vi "LinkNodes.vi"(0 "Parent in":refnum<data-value>, 5 "Child in":refnum<data-value>, 7 "ParentLinkInfo":T1, 9 "ChildLinkInfo":T1, 11 "error in (no error)":errorcluster) -> (4 "Parent out":refnum<data-value>, 6 "Child out":refnum<data-value>, 15 "error out":errorcluster)   [LabVIEW 2014, in "MultiTree.lvlib" / "MultiTree.lvclass"]
uses:
  <userlib>/AdvancedDataStructures/ClassBased/MultiTree/MultiTree.lvclass
  <userlib>/AdvancedDataStructures/ClassBased/MultiTreeNode/MultiTreeNode.lvclass
  <userlib>/AdvancedDataStructures/ClassBased/MultiTree/LinkInfo.ctl
  <userlib>/AdvancedDataStructures/ClassBased/MultiTreeNode/MultiTreeNode.lvclass/MultiTreeNode.ctl
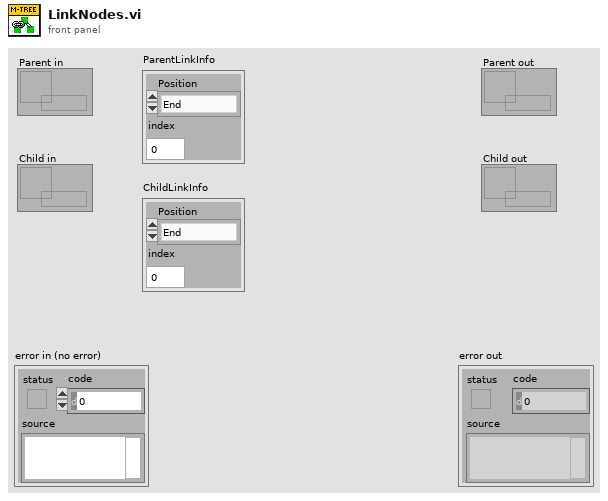
[diagram p1: front panel]
types:
  T1 = typedef "MultiTree.lvlib/MultiTree.lvclass/LinkInfo.ctl" = cluster{"Position":enum16{"End", "Front", "Index"}, "index":i32}
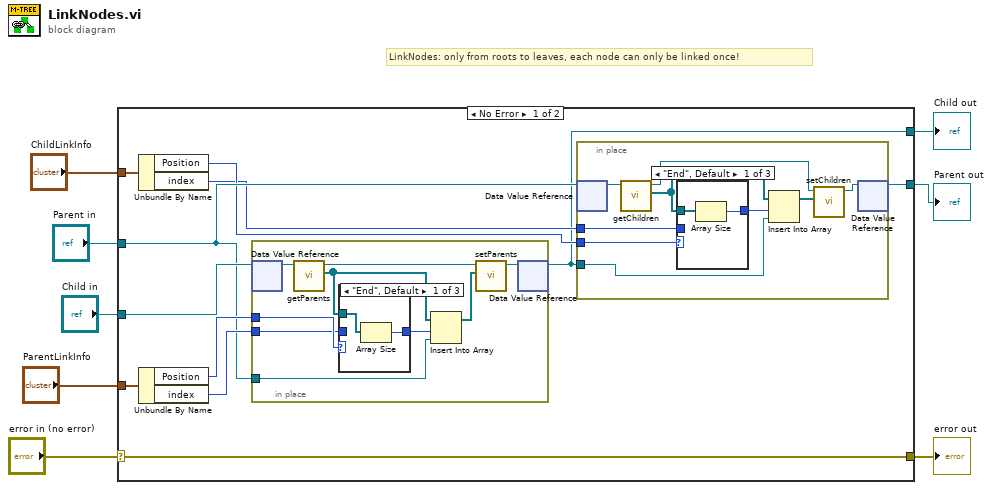
[diagram p0: block diagram]
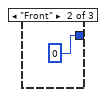
[diagram p2: hidden frame]
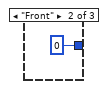
[diagram p4: hidden frame]
diagram:
  # "LinkNodes: only from roots to leaves, each node can only be linked once!"
  n1 = case shown="No Error" "error in (no error)" {
    selector: "error in (no error)" -> [w19 w48]
    tunnel: [w19 w48] -> w7
    tunnel: "Child in" -> [w15 w46]
    tunnel: [w10 w47] -> w4
    tunnel: "Parent in" -> [w13 w47]
    tunnel: [w9 w46] -> w3
    tunnel: "ParentLinkInfo" -> [w18 _]
    tunnel: "ChildLinkInfo" -> [w17 _]
    frame No Error {
      n2 = Unbundle By Name(w17) -> ("Position"=w12:enum16{"End", "Front", "Index"}, "index"=w11:i32)
      n3 = Unbundle By Name(w18) -> ("Position"=w16:enum16{"End", "Front", "Index"}, "index"=w14:i32)
      n4 = in-place {
        in-place-border: w16 -> [w41]
        in-place-border: w14 -> [w36]
        in-place-border: w13 -> [w33]
        n5 = in-place-dvr #1(w15) -> (w40:refnum<class "MultiTreeNode.lvclass">)  [unwired: 1 out]
        n6 = call <userlib>:"getParents.vi"("MultiTreeNode in"=w40) -> ("Parents"=w35:refnum<data-value>[], "MultiTreeNode out"=w39:refnum<class "MultiTreeNode.lvclass">)  [unwired: 8 in, 1 out]
        n7 = case shown="\"End\", Default" w41 {
          tunnel: [w42 0 w45] -> w34
          tunnel: w36 -> [_ _ w45]
          tunnel: w35 -> [w43 _ _]
          frame "End", Default {
            n8 = Array Size(array=w43) -> (size(s)=w42:i32)
          }
          frame "Front" {
          }
          frame "Index" {
          }
        }
        n9 = Insert Into Array(array=w35, index=w34, new element=w33) -> (w37:refnum<data-value>[])
        n10 = call <userlib>:"setParents.vi"("Parents"=w37, "MultiTreeNode in"=w39) -> ("MultiTreeNode out"=w38:refnum<class "MultiTreeNode.lvclass">)  [unwired: 8 in, 1 out]
        n11 = in-place-dvr #1(w38) -> (w9:refnum<data-value>)  [unwired: 1 out]
      }
      n12 = in-place {
        in-place-border: w12 -> [w28]
        in-place-border: w11 -> [w23]
        in-place-border: w9 -> [w20]
        n13 = in-place-dvr #2(w13) -> (w27:refnum<class "MultiTreeNode.lvclass">)  [unwired: 1 out]
        n14 = call <userlib>:"getChildren.vi"("MultiTreeNode in"=w27) -> ("Children"=w22:refnum<data-value>[], "MultiTreeNode out"=w26:refnum<class "MultiTreeNode.lvclass">)  [unwired: 8 in, 1 out]
        n15 = case shown="\"End\", Default" w28 {
          tunnel: [w29 0 w32] -> w21
          tunnel: w23 -> [_ _ w32]
          tunnel: w22 -> [w30 _ _]
          frame "End", Default {
            n16 = Array Size(array=w30) -> (size(s)=w29:i32)
          }
          frame "Front" {
          }
          frame "Index" {
          }
        }
        n17 = Insert Into Array(array=w22, index=w21, new element=w20) -> (w24:refnum<data-value>[])
        n18 = call <userlib>:"setChildren.vi"("Children"=w24, "MultiTreeNode in"=w26) -> ("MultiTreeNode out"=w25:refnum<class "MultiTreeNode.lvclass">)  [unwired: 8 in, 1 out]
        n19 = in-place-dvr #2(w25) -> (w10:refnum<data-value>)  [unwired: 1 out]
      }
    }
    frame Error {
    }
  }
  "error out" <- w7
  "Parent out" <- w4
  "Child out" <- w3
